vi "North.vi"(9 "Spheres in":cluster{i32, i32}[](array[cluster]), 10 "Cubes":cluster{i32, i32}[](array[cluster]), 11 "Northmost":i32) -> (1 "Spheres out":cluster{i32, i32}[](array[cluster]))   [LabVIEW 2023, in "d14.lvlib"]
uses:
  d14.lvlib
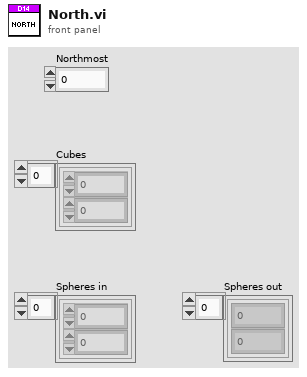
[diagram p1: front panel]
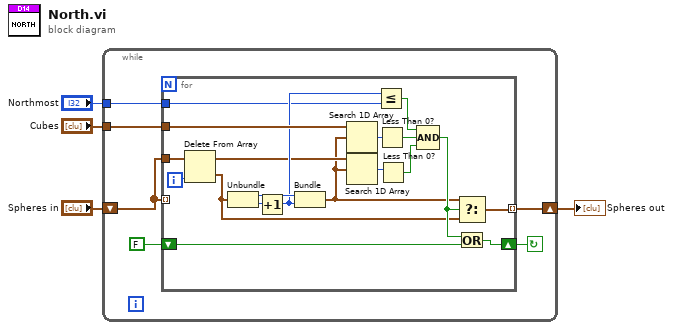
[diagram p0: block diagram]
diagram:
  n1 = while {
    tunnel: "Cubes" -> [w10]
    shift-right: [w9] -> w4
    shift-left: "Spheres in" -> [w5]
    tunnel: "Northmost" -> [w8]
    stop <- w6 continue-if-true
    n2 = for {
      tunnel: w10 -> [w29]
      tunnel: w5 -> [_] mode=indexing
      tunnel: [w25] -> w9 mode=indexing
      tunnel: w8 -> [w23]
      shift-right: [w18] -> w6
      shift-left: FALSE ("x .and. y?") -> [w19]
      tunnel: w5 -> [w17]
      i -> [w15]
      n3 = Delete From Array(array=w17, index=w15) -> (deleted portion=w14:cluster{i32, i32}, array with subset deleted=w16:cluster{i32, i32}[])  [unwired: 1 in]
      n4 = Unbundle(w14) -> (w27:i32, w28:i32)
      n5 = Increment(x=w28) -> (x+1=w24:i32)
      n6 = Bundle(w27, w24) -> (w13:cluster{i32, i32})  [unwired: 1 in]
      n7 = Search 1D Array(1D array=w29, element=w13) -> (index of element=w26:i32)  [unwired: 1 in]
      n8 = Search 1D Array(1D array=w16, element=w13) -> (index of element=w12:i32)  [unwired: 1 in]
      n9 = Less Or Equal?(x=w24, y=w23) -> (x <= y?=w22:bool)
      n10 = Less Than 0?(x=w26) -> (x < 0?=w21:bool)
      n11 = Less Than 0?(x=w12) -> (x < 0?=w11:bool)
      n12 = Compound Arithmetic op=AND(w22, w21, w11) -> (w20:bool)
      n13 = Select(t=w13, s=w20, f=w14) -> (s? t:f=w25:cluster{i32, i32})
      n14 = Or(x=w20, y=w19) -> (x .or. y?=w18:bool)
    }
  }
  "Spheres out" <- w4
